vi "Read Abs_Waveform.vi"(8 "error in (no error)":errorcluster, 11 "Measure Freq in":refnum<class "Measure Waveform.lvclass">) -> (0 "error out":errorcluster, 2 "Abs_Waveform.lvclass":refnum<class "Abs_Waveform.lvclass">, 3 "Measure Freq out":refnum<class "Measure Waveform.lvclass">)   [LabVIEW 2021, in "Measure Waveform.lvclass"]
uses:
  Measure Waveform.lvclass
  <vilib>/TSA/Abstract Data Classes/Abs_Types/Waveform/Abs_Waveform.lvclass
  Measure Waveform.lvclass/Measure Waveform.ctl
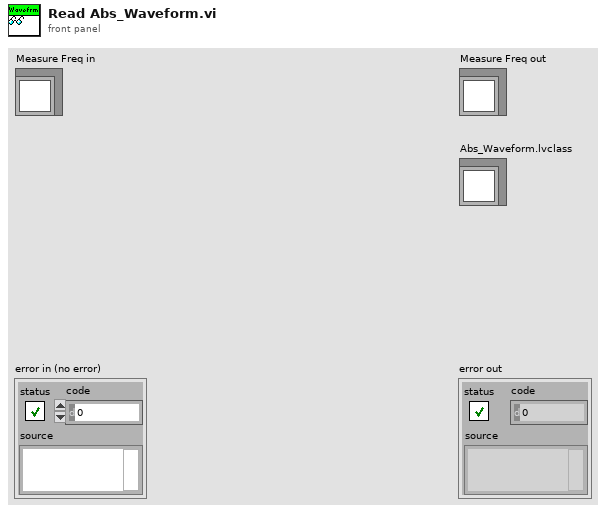
[diagram p1: front panel]
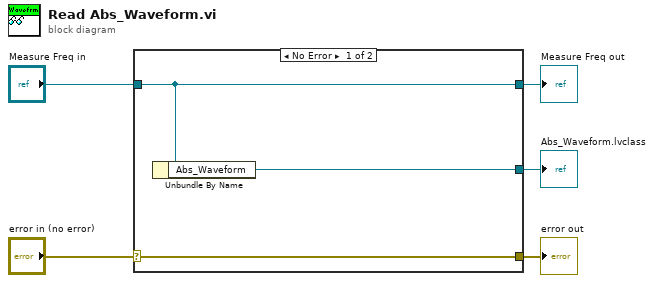
[diagram p0: block diagram]
diagram:
  n1 = case shown="No Error" "error in (no error)" {
    selector: "error in (no error)" -> [w8 w9]
    tunnel: [w8 w9] -> w4
    tunnel: [w7 w10] -> w2
    tunnel: "Measure Freq in" -> [w7 w10]
    tunnel: [w6 _] -> w1
    frame No Error {
      n2 = Unbundle By Name(w7) -> ("Abs_Waveform"=w6:refnum<class "Abs_Waveform.lvclass">)
    }
    frame Error {
    }
  }
  "error out" <- w4
  "Measure Freq out" <- w2
  "Abs_Waveform.lvclass" <- w1
